vi "pdw 2 graph.vi"(9 "color plate":T14, 10 "PDW":cluster{"PDW":T12[], "Ton":dbl[]} {"PDW"."frequency shift" format="%#_12f"}, 11 "secnario config":T1 {"mode" scale=0.0..2.0; "RF gain" min=0 max=31 step=1; "niUsrpRio Session (out)"."Daughterboard Clock Rate" format="%#.3pHz"; "niUsrpRio Session (out)"."FPGA Data Clock Rate" format="%#.3pHz"; "niUsrpRio Session (out)"."Data Clock Rate" format="%#.3pHz"; "niUsrpRio Session (out)"."Characterization Data"."Frequencies [Hz]" format="%#_6p"; "niUsrpRio Session (out)"."EEPROM Characterization Header"."Pointer to Device Data Header" format="%x"; "niUsrpRio Session (out)"."EEPROM Characterization Header"."Checksum" format="%x"; "niUsrpRio Session (out)"."Device Data Header"."Pointer to Characterization Data" format="%x"; "niUsrpRio Session (out)"."Device Data Header"."Checksum" format="%x"; "niUsrpRio Session (out)"."EEPROM Header"."Pointer to User Header" format="%x"; "niUsrpRio Session (out)"."EEPROM Header"."Pointer to Factory Header" format="%x"; "niUsrpRio Session (out)"."EEPROM Header"."Product Code" format="%x"; "niUsrpRio Session (out)"."EEPROM Header"."Checksum" format="%x"; "center frequency (Hz)" format="%#.8p"; "buffer size" step=512}) -> (2 "color":u32[](array[numeric]), 3 "graph":cluster{dbl[], dbl[]}[](array[cluster]))   [LabVIEW 2021]
uses:
  pdw.ctl
  mode_type.ctl
  secnario config.ctl
  <vilib>/userdefined/High Color/nirio_resource_hc.ctl
  <instrlib>/niUsrpRio/Config/v1/Host/Public/niUsrpRio Session.ctl
  <instrlib>/_niInstr/Register Bus/v0/Host/Public/Register Bus Session.ctl
  <instrlib>/_niInstr/Register Bus/v0/Host/Private/Session Data.ctl
  <instrlib>/niUsrpRio/Config/v1/Host/Private/DB Queue Reference.ctl
  <instrlib>/niUsrpRio/Config/v1/Host/Private/Daughterboard Data.ctl
  <instrlib>/niUsrpRio/Config/v1/Host/Private/ATR state data.ctl
  <instrlib>/niUsrpRio/Config/v1/Host/Private/Antenna Configuration.ctl
  <instrlib>/niUsrpRio/Config/v1/Host/Private/CPLD Power Mode.ctl
  <instrlib>/niUsrpRio/Config/v1/Host/Public/EEPROM Header.ctl
  <instrlib>/niUsrpRio/Config/v1/Host/Public/EEPROM Device Data Header.ctl
  <instrlib>/niUsrpRio/Config/v1/Host/Public/EEPROM Characterization Header.ctl
  <instrlib>/niUsrpRio/Config/v1/Host/Public/Characterization Data.ctl
  <instrlib>/niUsrpRio/Config/v1/Host/Public/IQ Imbalance.ctl
  <instrlib>/_niInstr/Register Bus/v0/Host/niInstr Register Bus v0 Host.lvlib
  <instrlib>/niUsrpRio/Config/v1/Host/niUsrpRio Config v1 Host.lvlib
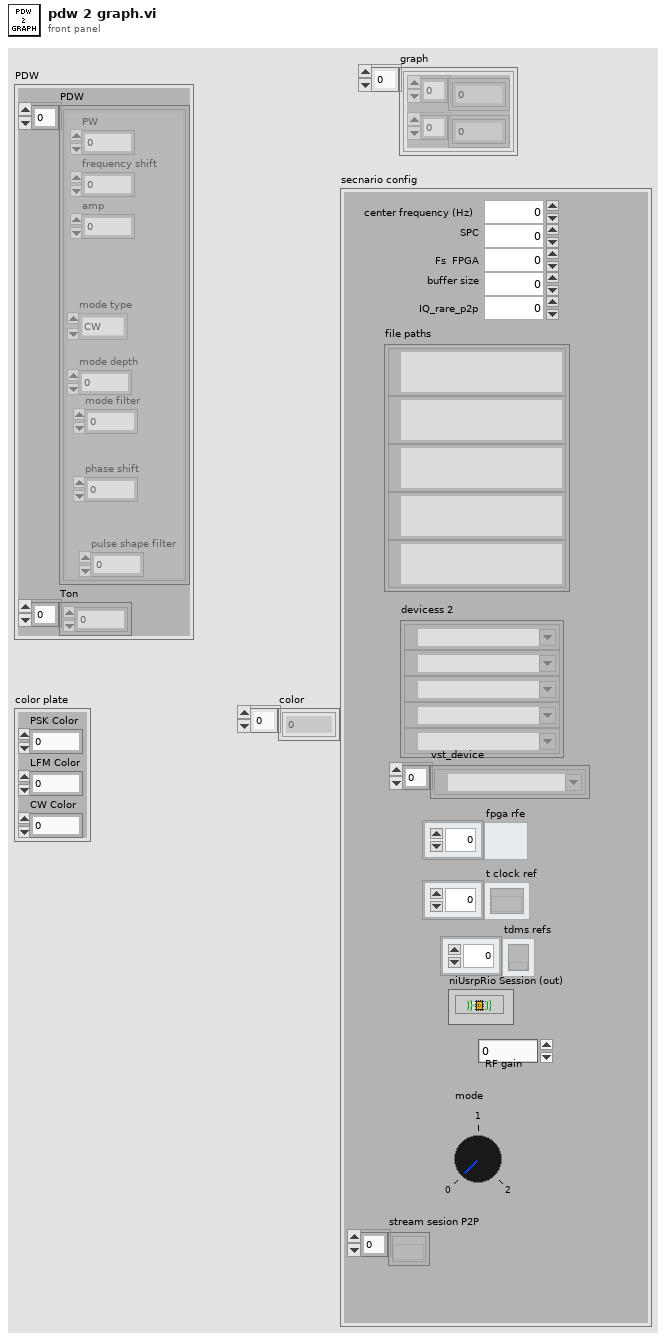
[diagram p1: front panel]
types:
  T1 = typedef "secnario config.ctl" = cluster{"devicess 2":T2[], "file paths":path[], "buffer size":u32, "Fs  FPGA":dbl, "SPC":dbl, "center frequency (Hz) ":dbl, "t clock ref":refnum<k20>[], "fpga rfe":refnum<k20>[], "tdms refs":refnum<k34>[], "niUsrpRio Session (out)":T3, "RF gain ":i32, "mode":u8, "vst_device":refnum<k15>[], "IQ_rare_p2p":dbl, "stream sesion P2P":refnum<k20>[]}
  T2 = typedef "nirio_resource_hc.ctl" = tag
  T3 = typedef "niUsrpRio Config v1 Host.lvlib/niUsrpRio Session.ctl" = cluster{"FPGA Interface":refnum<k20>, "RIO Interface Number":u32, "Data Clock Rate":u32, "FPGA Data Clock Rate":u32, "Global Settings Register Bus":T4, "Radio 0 Settings Register Bus":T4, "Radio 1 Settings Register Bus":T4, "Radio Settings Bus Semaphore":T5, "DB Queues":T6[], "Characterization Data Valid?":bool, "EEPROM Header":T7, "Device Data Header":T8, "EEPROM Characterization Header":T9, "Characterization Data":T10[], "FPGA Current Version":u32, "FPGA Oldest Compatible Version":u32, "Fixed Logic Current Version":u32, "Fixed Logic Oldest Compatible Version":u32, "FPGA Radio Settings Bus Current Version":u32, "FPGA Radio Settings Bus Oldest Compatible Version":u32, "FPGA Board Config Current Version":u32, "FPGA Board Config Oldest Compatible Version":u32, "Daughterboard Clock Rate":u32, "daughterboard configuration session handles":u64[]}
  T4 = typedef "niInstr Register Bus v0 Host.lvlib/Register Bus Session.ctl" = refnum<queue>
  T5 = typedef "Semaphore RefNum" = refnum<k1>
  T6 = typedef "niUsrpRio Config v1 Host.lvlib/DB Queue Reference.ctl" = refnum<queue>
  T7 = typedef "niUsrpRio Config v1 Host.lvlib/EEPROM Header.ctl" = cluster{"Checksum":u32, "Product Code":u16, "Hardware Current Version":u16, "Hardware Oldest Compatible Version":u16, "EEPROM Map Current Version":u16, "EEPROM Map Oldest Compatible Version":u16, "User Password":string, "Pointer to Factory Header":u32, "Pointer to User Header":u32, "Recommended Interval":u16, "Number of Reserved Bytes":i32, "Number of Daughterboards":u8, "Daughterboard IDs":u16[], "Daughterboard Serial Numbers":string[]}
  T8 = typedef "niUsrpRio Config v1 Host.lvlib/EEPROM Device Data Header.ctl" = cluster{"Checksum":u32, "Number of Channels":u8, "Number of Gain Settings":u16[], "Pointer to Characterization Data":u32[], "Number of Reserved Bytes":i32, "Number of Frequencies":u16[]}
  T9 = typedef "niUsrpRio Config v1 Host.lvlib/EEPROM Characterization Header.ctl" = cluster{"Checksum":u32, "Date":timestamp, "Temperature":sgl, "Misc. Info":string, "Pointer to Device Data Header":u32, "Number of Reserved Bytes":i32}
  T10 = typedef "niUsrpRio Config v1 Host.lvlib/Characterization Data.ctl" = cluster{"Gains[dB]":dbl[], "Frequencies [Hz]":dbl[], "IQ Imbalance Table":T11[], "Measured Gains[dB]":dbl[][]}
  T11 = typedef "niUsrpRio Config v1 Host.lvlib/IQ Imbalance.ctl" = cluster{"Gain Imbalance [linear]":dbl, "Phase Imbalance [radians]":dbl, "Offset":cdb}
  T12 = typedef "pdw.ctl" = cluster{"PW":u32, "frequency shift":fxp<+/-,48,0>, "amp":fxp<+/-,18,1>, "mode type":T13, "mode depth":u32, "mode filter":u8, "phase shift":fxp<+/-,16,1>, "pulse shape filter":u8}
  T13 = typedef "mode_type.ctl" = enum8{"CW", "NC - CW", "NC - cw", "LFM", "BPSK", "QPSK"}
  T14 = cluster{"PSK Color":u32, "LFM Color":u32, "CW Color":u32}
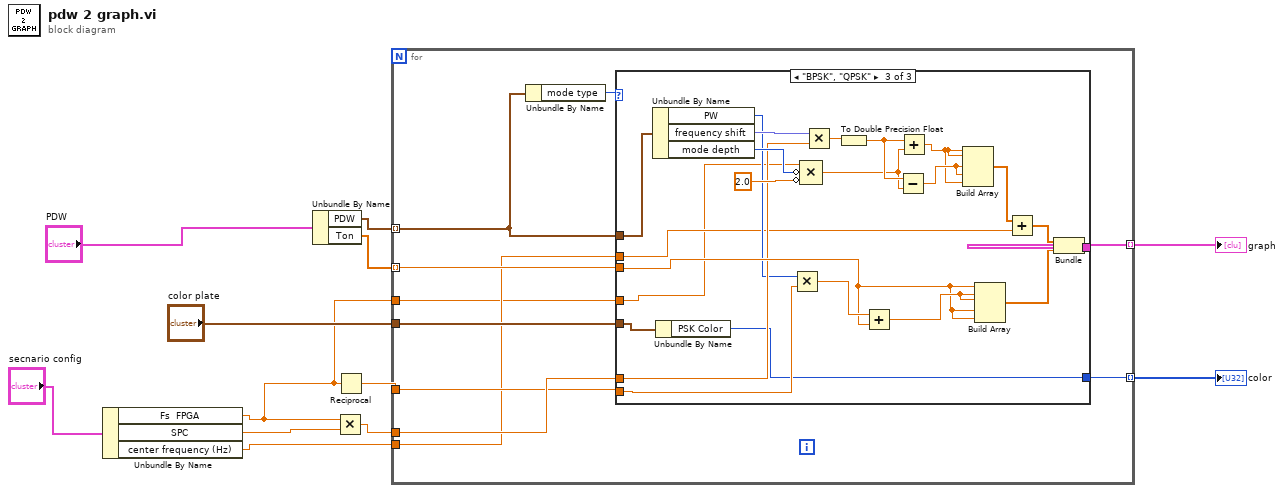
[diagram p0: block diagram]
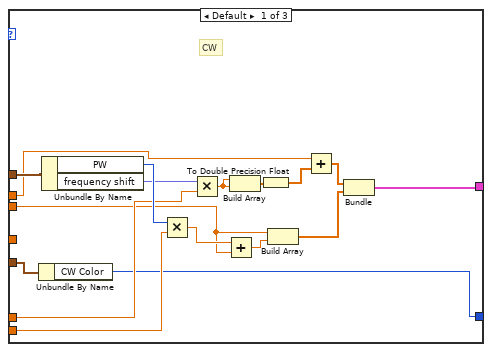
[diagram p2: hidden frame]
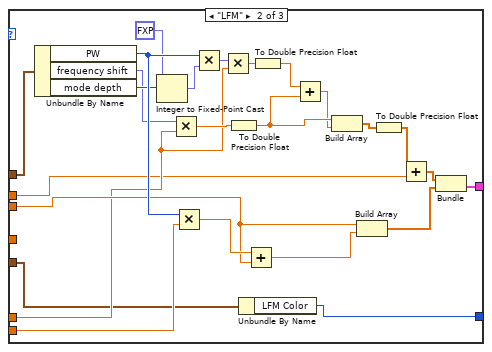
[diagram p3: hidden frame]
diagram:
  n1 = Unbundle By Name("secnario config") -> ("Fs  FPGA"=w1:dbl, "SPC"=w3:dbl, "center frequency (Hz)"=w2:dbl)
  n2 = Unbundle By Name("PDW") -> ("PDW"=w10:T12[], "Ton"=w11:dbl[])
  n3 = Multiply(x=w1, y=w3) -> (x*y=w8:dbl)
  n4 = Reciprocal(x=w1) -> (1/x=w5:dbl)
  n5 = for {
    tunnel: w8 -> [w21]
    tunnel: w5 -> [w20]
    tunnel: [w19] -> w6 mode=indexing
    tunnel: [w18] -> w7 mode=indexing
    tunnel: w10 -> [w17] mode=indexing
    tunnel: w11 -> [w16] mode=indexing
    tunnel: "color plate" -> [w15]
    tunnel: w2 -> [w14]
    tunnel: w1 -> [w13]
    n6 = Unbundle By Name(w17) -> ("mode type"=w22:T13)
    n7 = case shown="\"BPSK\", \"QPSK\"" w22 {
      tunnel: w16 -> [w29 w57 w82]
      tunnel: w17 -> [w39 w60 w84]
      tunnel: w21 -> [w36 w49 w79]
      tunnel: w20 -> [w35 w61 w85]
      tunnel: [w33 w62 w71] -> w19
      tunnel: [w24 w41 w67] -> w18
      tunnel: w15 -> [w25 w42 w68]
      tunnel: w14 -> [w23 w40 w66]
      tunnel: w13 -> [_ _ w65]
      frame Default {
        # "CW"
        n8 = Unbundle By Name(w25) -> ("CW Color"=w24:u32)
        n9 = Unbundle By Name(w39) -> ("PW"=w38:u32, "frequency shift"=w37:fxp<+/-,48,0>)
        n10 = Multiply(x=w38, y=w35) -> (x*y=w30:dbl)
        n11 = Multiply(x=w37, y=w36) -> (x*y=w34:dbl)
        n12 = Add(x=w30, y=w29) -> (x+y=w28:dbl)
        n13 = Build Array(w34, w34) -> (w31:dbl[])
        n14 = To Double Precision Float(number=w31) -> (double precision float=w27:dbl[])
        n15 = Build Array(w29, w28) -> (w32:dbl[])
        n16 = Add(x=w23, y=w27) -> (x+y=w26:dbl[])
        n17 = Bundle(w26, w32) -> (w33:cluster{dbl[], dbl[]})  [unwired: 1 in]
      }
      frame "LFM" {
        n18 = Unbundle By Name(w60) -> ("PW"=w59:u32, "frequency shift"=w51:fxp<+/-,48,0>, "mode depth"=w54:u32)
        n19 = Integer to Fixed-Point Cast(fixed-point type=fxp<+,32,-16> 0.0, integer=w54) -> (fixed-point=w50:fxp<+,32,-16>)
        n20 = Multiply(x=w51, y=w49) -> (x*y=w52:dbl)
        n21 = Multiply(x=w59, y=w61) -> (x*y=w58:dbl)
        n22 = Multiply(x=w59, y=w50) -> (x*y=w48:fxp<+,64,16>)
        n23 = Multiply(x=w48, y=w49) -> (x*y=w53:dbl)
        n24 = To Double Precision Float(number=w52) -> (double precision float=w47:dbl)
        n25 = Unbundle By Name(w42) -> ("LFM Color"=w41:u32)
        n26 = Add(x=w58, y=w57) -> (x+y=w56:dbl)
        n27 = To Double Precision Float(number=w53) -> (double precision float=w46:dbl)
        n28 = Add(x=w46, y=w47) -> (x+y=w45:dbl)
        n29 = Build Array(w47, w45) -> (w63:dbl[])
        n30 = Build Array(w57, w56) -> (w64:dbl[])
        n31 = To Double Precision Float(number=w63) -> (double precision float=w44:dbl[])
        n32 = Add(x=w44, y=w40) -> (x+y=w43:dbl[])
        n33 = Bundle(w43, w64) -> (w62:cluster{dbl[], dbl[]})  [unwired: 1 in]
      }
      frame "BPSK", "QPSK" {
        n34 = Unbundle By Name(w84) -> ("PW"=w76:u32, "frequency shift"=w78:fxp<+/-,48,0>, "mode depth"=w81:u32)
        n35 = Unbundle By Name(w68) -> ("PSK Color"=w67:u32)
        n36 = Multiply(x=w76, y=w85) -> (x*y=w86:dbl)
        n37 = Compound Arithmetic op=MULTIPLY(w65, invert w81, invert 2.0 ("value")) -> (w74:dbl)
        n38 = Multiply(x=w78, y=w79) -> (x*y=w77:dbl)
        n39 = To Double Precision Float(number=w77) -> (double precision float=w75:dbl)
        n40 = Add(x=w86, y=w82) -> (x+y=w83:dbl)
        n41 = Subtract(x=w75, y=w74) -> (x-y=w73:dbl)
        n42 = Add(x=w75, y=w74) -> (x+y=w72:dbl)
        n43 = Build Array(w72, w72, w73, w73, w72) -> (w70:dbl[])
        n44 = Build Array(w82, w83, w83, w82, w82) -> (w87:dbl[])
        n45 = Add(x=w70, y=w66) -> (x+y=w69:dbl[])
        n46 = Bundle(w69, w87) -> (w71:cluster{dbl[], dbl[]})  [unwired: 1 in]
      }
    }
  }
  "color" <- w7
  "graph" <- w6
